vi "pythonEmbedTest.vi"() -> ()   [LabVIEW 2017]
uses:
  dll/wormUtilities/x64/Release/wormUtilities.dll
panel:
  out "return type":dbl
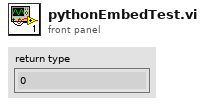
[diagram p1: front panel]
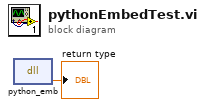
[diagram p0: block diagram]
diagram:
  n1 = dll-call lib="C:/Users/francesco/dev/pump-probe/dll/wormUtilities/x64/Release/wormUtilities.dll" fn="python_emb"() -> ("return type"=→"return type":dbl)  [unwired: 3 in, 2 out]
